vi "Read Input Registers.vi"(8 "error in":errorcluster, 9 "number of registers":u16, 10 "starting address":u16, 11 "device data model in":refnum<class "Standard Data Model.lvclass">) -> (0 "error out":errorcluster, 2 "data":u16[](array[numeric]), 3 "device data model out":refnum<class "Standard Data Model.lvclass">)   [LabVIEW 2021, in "Standard Data Model.lvclass"]
doc: "Reads N input registers from the device model, starting at register M."
uses:
  Standard Data Model.lvclass
  Standard Data Model.lvclass/Standard Data Model.ctl
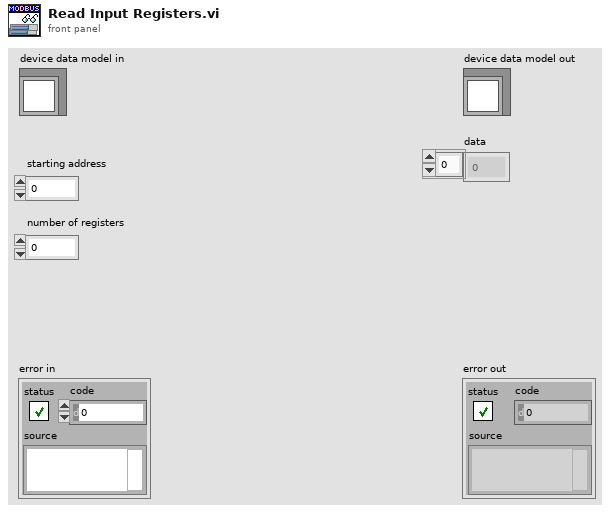
[diagram p1: front panel]
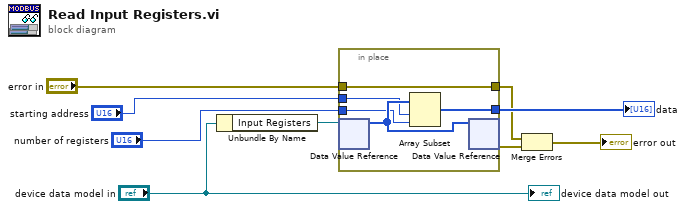
[diagram p0: block diagram]
diagram:
  n1 = Unbundle By Name("device data model in") -> ("Input Registers"=w7:refnum<data-value>)
  n2 = in-place {
    in-place-border: "error in" -> [w14]
    in-place-border: [w14] -> w1
    in-place-border: [w12] -> w8
    in-place-border: "starting address" -> [w11]
    in-place-border: "number of registers" -> [w10]
    n3 = in-place-dvr #1(w7) -> (w13:u16[])  [unwired: 1 out]
    n4 = Array Subset(array=w13, index=w11, length=w10) -> (w12:u16[])
    n5 = in-place-dvr #1(w13) -> (w2:errorcluster)  [unwired: 1 out]
  }
  "data" <- w8
  n6 = Merge Errors(w1, w2) -> (→"error out":errorcluster)
  "device data model out" <- "device data model in"
